vi "Alicat Simplified Driver Example_Multiple Devices.vi"() -> ()   [LabVIEW 2019]
doc: "Simplified example program for initializing the COM port, determining the data frame of up to 26 Alicats, acquiring the data of the same number of Alicats, and displaying the data of the one with the selected unit ID.\n\nThis is a slightly more feature rich version of the Alicat Simplified Driver Example, and contains an example of a method for interfacing with up to 26 Alicats on a single COM port by means of for loops with shift registers to handle sequential commands to each included Alicat.\n\nIf coding for multiple Alicats on a single COM port without the use of for loops with shift registers, ensure that each Alicat command is executed sequentially. Alicat's RS-232/485 does not work if multiple devices are responding simultaneously."
panel:
  out "Meas. Data (for active device)":T1
  in  "Display Data\nFor Device:":u16(ring) items=["A"]
  in  "Device ID's \nto Include:":T2
  in  "Minimum time between \nreadings [ms] (all units)":u32
  out "Elapsed Time [ms]\n(all units)":dbl caption="Elapsed Time (s)"
  in  "End Program":bool
  out "Error Text":string
  out "Error Present":bool
  out "Range Exceeded":bool
  in  "COM Port Settings":T3={"Baud Rate"=enum."19200", "VISA Sesssion In"="COM1"}
  # "Totalizer Timer"
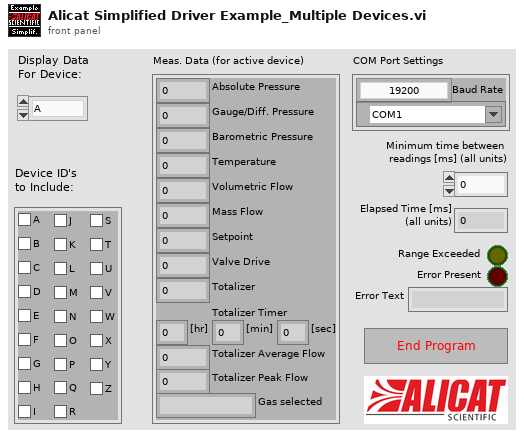
[diagram p1: front panel]
types:
  T1 = cluster{"Absolute Pressure":dbl, "Gauge/Diff. Pressure":dbl, "Barometric Pressure":dbl, "Temperature":dbl, "Volumetric Flow":dbl, "Mass Flow":dbl, "Setpoint":dbl, "Valve Drive":dbl, "Totalizer":dbl, "[hr]":dbl, "[min]":dbl, "[sec]":dbl, "Totalizer Average Flow":dbl, "Totalizer Peak Flow":dbl, "Gas selected":string}
  T2 = cluster{"A":bool, "B":bool, "C":bool, "D":bool, "E":bool, "F":bool, "G":bool, "H":bool, "I":bool, "J":bool, "K":bool, "L":bool, "M":bool, "N":bool, "O":bool, "P":bool, "Q":bool, "R":bool, "S":bool, "T":bool, "U":bool, "V":bool, "W":bool, "X":bool, "Y":bool, "Z":bool}
  T3 = cluster{"Baud Rate":enum8{"2400", "9600", "19200", "38400", "57600", "115200", "Unknown"}, "VISA Sesssion In":refnum<visa-resource-name>}
  T4 = cluster{"Unit ID":string, "Baud Rate":enum8{"2400", "9600", "19200", "38400", "57600", "115200", "Unknown"}, "VISA Sesssion In":refnum<visa-resource-name>}
  T5 = enum8{"2400", "9600", "19200", "38400", "57600", "115200", "Unknown"}
  T6 = typedef "Data Frame.ctl" = cluster{"Absolute Pressure":bool, "Gauge/Diff. Pressure":bool, "Barometric Pressure":bool, "Temperature":bool, "Volumetric":bool, "Mass":bool, "Setpoint":bool, "Valve Drive":bool, "Totalizer":bool, "Totalizer Timer":bool, "Totalizer Average Flow":bool, "Totalizer Peak Flow":bool, "Gas Selected":bool, "Tot. Timer Format":u16}
  T7 = typedef "Data Cluster.ctl" = cluster{"Absolute Pressure":dbl, "Gauge/Diff. Pressure":dbl, "Barometric Pressure":dbl, "Temperature":dbl, "Volumetric Flow":dbl, "Mass Flow":dbl, "Setpoint":dbl, "Valve Drive":dbl, "Totalizer":dbl, "[hr]":dbl, "[min]":dbl, "[sec]":dbl, "Totalizer Average Flow":dbl, "Totalizer Peak Flow":dbl, "Gas selected":string}
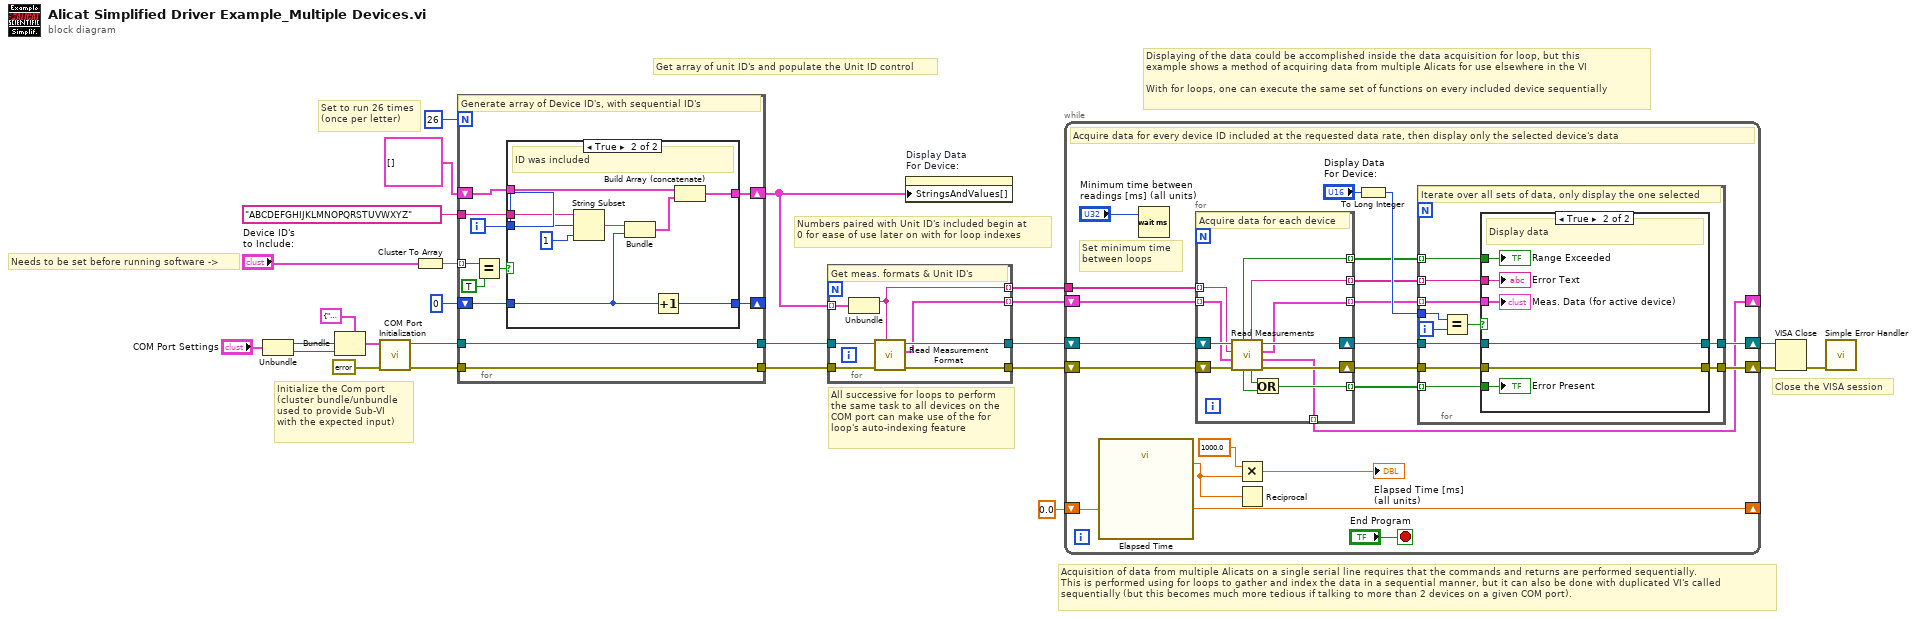
[diagram p0: block diagram]
diagram:
  # "All successive for loops to perform\nthe same task to all devices on the\nCOM port can make use of the for\nloop's auto-indexing feature"
  # "Set to run 26 times\n(once per letter)"
  # "Acquisition of data from multiple Alicats on a single serial line requires that the commands and returns are performed sequentially.\nThis is performed using for loops to gather and index the data in a sequential manner, but it can also be done with duplicated VI's called\nsequentially (but this becomes much more tedious if talking to more than 2 devices on a given COM port)."
  # "Numbers paired with Unit ID's included begin at\n0 for ease of use later on with for loop indexes"
  # "Displaying of the data could be accomplished inside the data acquisition for loop, but this\nexample shows a method of acquiring data from multiple Alicats for use elsewhere in the VI\n\nWith for loops, one can execute the same set of functions on every included device sequentially"
  # "Get array of unit ID's and populate the Unit ID control"
  # "Needs to be set before running software ->"
  # "Close the VISA session"
  # "Initialize the Com port\n(cluster bundle/unbundle\nused to provide Sub-VI \nwith the expected input)"
  n1 = Unbundle("COM Port Settings") -> ("Baud Rate"=w18:T5, "VISA Sesssion In"=w17:refnum<visa-resource-name>)
  n2 = Bundle(cluster=T4 {"Unit ID"="A", "Baud Rate"=enum."19200", "VISA Sesssion In"="COM1"} ("Communication Settings"), "Baud Rate"=w18, "VISA Sesssion In"=w17) -> (w16:T4)  [unwired: 1 in]
  n3 = call "COM Port Initialization.vi"("error in (no error)"=errorcluster {"status"=FALSE, "code"=0, "source"=""}, "Communication Settings"=w16) -> ("error out"=w9:errorcluster, "VISA Session Out"=w8:refnum<visa-resource-name>)  [unwired: 8 in]
  n4 = Cluster To Array(cluster="Device ID's \nto Include:") -> (array=w12:bool[])
  n5 = for {
    N: 26 -> [_]
    tunnel: "ABCDEFGHIJKLMNOPQRSTUVWXYZ" -> [w36]
    tunnel: w12 -> [w29] mode=indexing
    shift-right: [w28] -> _
    shift-left: u16 0 ("length (rest)") -> [w34]
    shift-right: [w33] -> w5
    shift-left: cluster{string, u16}[] [] -> [w32]
    tunnel: w9 -> [w27]
    tunnel: w8 -> [w26]
    tunnel: [w27] -> w6
    tunnel: [w26] -> w7
    i -> [w35]
    # "Generate array of Device ID's, with sequential ID's"
    n6 = Equal?(x=w29, y=TRUE) -> (x = y?=w31:bool)
    n7 = case shown="True" w31 {
      tunnel: w36 -> [_ w47]
      tunnel: w35 -> [_ w46]
      tunnel: w34 -> [w37 w39]
      tunnel: [w38 w42] -> w33
      tunnel: w32 -> [w38 w40]
      tunnel: [w37 w43] -> w28
      frame False {
        # "ID was not included"
      }
      frame True {
        # "ID was included"
        n8 = String Subset(string=w47, offset (0)=w46, length (rest)=1 ("length (rest)")) -> (substring=w44:string)
        n9 = Bundle(w44, "length (rest)"=w39) -> (w41:cluster{string, "length (rest)":u16})  [unwired: 1 in]
        n10 = Increment(x=w39) -> (x+1=w43:u16)
        n11 = Build Array (concatenate)(w40, w41) -> (w42:cluster{string, "length (rest)":u16}[])
      }
    }
  }
  n12 = for {
    tunnel: w7 -> [w53]
    tunnel: [w51] -> w2
    tunnel: w6 -> [w54]
    tunnel: [w52] -> w1
    tunnel: w5 -> [w49] mode=indexing
    tunnel: [w50] -> w4 mode=indexing
    tunnel: [w48] -> w3 mode=indexing
    # "Get meas. formats & Unit ID's"
    n13 = Unbundle(w49) -> (w48:string)  [unwired: 1 out]
    n14 = call "Read Measurement Format.vi"("Unit ID (A)"=w48, "error in"=w54, "VISA Session In"=w53) -> ("error out"=w52:errorcluster, "Data Frame Format"=w50:T6, "VISA Session Out"=w51:refnum<visa-resource-name>)  [unwired: 6 in]
  }
  n15 = property on="Display Data\nFor Device:" class="Ring (strict)"("StringsAndValues[]"=w5) -> ()  [unwired: 2 in, 2 out]
  n16 = while {
    shift-right: [w73] -> _
    shift-left: 0.0 ("Set Start Time (s)") -> [w76]
    shift-right: [w64] -> w21
    shift-left: w1 -> [w75]
    shift-right: [w62] -> w22
    shift-left: w2 -> [w74]
    tunnel: w3 -> [w66]
    shift-right: [w55] -> _
    shift-left: w4 -> [w67]
    stop <- "End Program" stop-if-true
    # "Set minimum time\nbetween loops"
    # "Acquire data for every device ID included at the requested data rate, then display only the selected device's data"
    n17 = call "Elapsed Time"("Set Start Time (s)"=w76) -> ("Get Start Time (s)"=w73:dbl, "Elapsed Time (s)"=w69:dbl)  [unwired: 11 in, 6 out]
    n18 = Wait (ms)(milliseconds to wait="Minimum time between \nreadings [ms] (all units)") -> ()  [unwired: 1 out]
    n19 = for {
      shift-right: [w105] -> w65
      shift-left: w75 -> [w108]
      shift-right: [w106] -> w63
      shift-left: w74 -> [w107]
      tunnel: w67 -> [w102] mode=indexing
      tunnel: w66 -> [w101] mode=indexing
      tunnel: [w100] -> w61 mode=indexing
      tunnel: [w99] -> w58 mode=indexing
      tunnel: [w98] -> w57 mode=indexing
      tunnel: [w97] -> w56 mode=indexing
      tunnel: [w96] -> w55 mode=indexing
      # "Acquire data for each device"
      n20 = call "Read Measurements.vi"("error in"=w108, "Data Frame Format In"=w102, "Unit ID (A)"=w101, "VISA Session In"=w107) -> ("error out"=w105:errorcluster, "Data Frame Format Out"=w96:T6, "Data Cluster"=w99:T7, "VISA Session Out"=w106:refnum<visa-resource-name>, "Unknown Dataframe Info"=w104:bool, "Error/Overrange/Unknown String"=w98:string, "Error Present"=w103:bool, "Range Exceeded"=w97:bool)
      n21 = Or(x=w104, y=w103) -> (x .or. y?=w100:bool)
    }
    n22 = Multiply(x=1000.0 ("y"), y=w69) -> (x*y=→"Elapsed Time [ms]\n(all units)":dbl)
    n23 = Reciprocal(x=w69) -> ()  [unwired: 1 out]
    n24 = To Long Integer(number="Display Data\nFor Device:") -> (32bit integer=w59:i32)
    n25 = for {
      tunnel: w65 -> [w79]
      tunnel: [w78] -> w64
      tunnel: w63 -> [w80]
      tunnel: [w77] -> w62
      tunnel: w61 -> [w85] mode=indexing
      tunnel: w59 -> [w87]
      tunnel: w58 -> [w84] mode=indexing
      tunnel: w57 -> [w83] mode=indexing
      tunnel: w56 -> [w82] mode=indexing
      i -> [w86]
      # "Iterate over all sets of data, only display the one selected"
      n26 = Equal?(x=w87, y=w86) -> (x = y?=w81:bool)
      n27 = case shown="True" w81 {
        tunnel: w85 -> [_ w95]
        tunnel: w84 -> [_ w90]
        tunnel: w83 -> [_ w94]
        tunnel: w82 -> [_ w93]
        tunnel: w80 -> [w89 w91]
        tunnel: w79 -> [w88 w92]
        tunnel: [w88 w92] -> w78
        tunnel: [w89 w91] -> w77
        frame False {
          # "Do nothing"
        }
        frame True {
          # "Display data"
          "Range Exceeded" <- w93
          "Error Present" <- w95
          "Error Text" <- w94
          "Meas. Data (for active device)" <- w90
        }
      }
    }
  }
  n28 = VISA Close(VISA resource name=w22, error in (no error)=w21) -> (error out=w23:errorcluster)
  n29 = call <vilib>:"Simple Error Handler.vi"("error in (no error)"=w23) -> ()  [unwired: 4 in, 5 out]
